vi "LSMcontroller_v66_improvedwfhandling.vi"() -> ()   [LabVIEW 2015] (continued)
                    n4209 = local read "Vy-max draw"() -> (w1158:dbl)
                    n4210 = local read "Vx-min draw"() -> (w1161:dbl)
                    n4211 = local read "Vx-max draw"() -> (w1160:dbl)
                    n4212 = local read "xpixels ref"() -> (w1157:i32)
                    n4213 = local read "ypixels ref"() -> (w1156:i32)
                    n4214 = local read "ROI Type"() -> (w1155:u16)
                    n4215 = local read "srateAODOtt"() -> (w1166:dbl)
                    n4216 = local read "# of frames"() -> (w1171:i32)
                    n4217 = local read "refreshtime"() -> (w1163:dbl)
                    n4218 = local read "Pel"() -> (w1154:dbl)
                    n4219 = local read "bin"() -> (w1169:dbl)
                    n4220 = local read "Override AI buffer"() -> (w1152:bool)
                    n4221 = local read "finite samples"() -> (w1178:bool)
                    n4222 = local read "srateAODOtt"() -> (w1165:dbl)
                    n4223 = local read "srateAODOtt"() -> (w1172:dbl)
                    n4224 = local read "continuous"() -> (w1177:bool)
                    n4225 = local read "Angle ref"() -> (w1162:dbl)
                    n4226 = local read "wavdet"() -> (w1179:bool)
                    n4227 = local read "Vx-ref"() -> (w1174:dbl)
                    n4228 = local read "Vy-ref"() -> (w1176:dbl)
                    n4229 = local read "avpp"() -> (w1175:i32)
                    n4230 = call "tt_timeandsamples.vi"("bin"=w1169, "refreshtime"=w1163, "srateAODOtt"=w1166, "tot#ofsamples"=w1171) -> ("refreshrate"=w1167:dbl, "refreshbuffer"=w1168:i32, "timetracecycles"=w1173:i32)  [unwired: 5 in]
                    n4231 = local read "bin"() -> (w1170:dbl)
                    n4232 = call "2pparameters.vi"("command"="get") -> ("params out"=w1182:T10)  [unwired: 1 in]
                    n4233 = Bundle By Name(cluster=w1182, "Drawing Mode"=w1155, "measpoints"=w1171, "tt_cycles"=w1173, "refreshbuffer"=w1168, "refreshrate"=w1167, "Vx-ref"=w1174, "Vy-ref"=w1176, "srate"=w1165, "finite"=w1178, "cont"=w1177, "wavdet"=w1179, "avpp"=w1175, "srateAODO"=w1172, "bufferAI"=w1168, "bin"=w1170, "Angle Img"=w1162, "Vxminref"=w1161, "Vxmaxref"=w1160, "Vyminref"=w1159, "Vymaxref"=w1158, "Xpixels Img"=w1157, "Ypixels Img"=w1156, "Pel"=w1154, "Vz-reset"=0.0, "AIoverride"=w1152, "type"="Timetrace") -> (w1180:T10)
                    n4234 = Reciprocal(x=w1167) -> (1/x=w1164:dbl)
                    n4235 = local write "refreshtime"(w1164) -> ()
                    n4236 = call "2pparameters.vi"("Params in"=w1180, "command"="set") -> ()  [unwired: 1 out]
                  }
                  frame "Lifetime (point)" {
                  }
                }
              }
              frame #1 {
                w1185 = FALSE ("wavdet")
                n4237 = call "2pparameters.vi"("command"="get") -> ("params out"=w1189:T10)  [unwired: 1 in]
                n4238 = Bundle By Name(cluster=w1189, "finite"=w1185, "cont"=w1185, "wavdet"=TRUE) -> (w1186:T10)
                n4239 = call "2pparameters.vi"("Params in"=w1186, "command"="set") -> ()  [unwired: 1 out]
              }
              frame #2 {
                n4240 = local read "Meastab"() -> (w1194:enum32{"X-Y Image", "Linescan", "Timetrace"})
                n4241 = property on="refwf" class="Ring (strict)"() -> ("RingText.Text"=w1197:string)  [unwired: 2 in, 2 out]
                n4242 = case shown="\"Timetrace\"" w1194 {
                  tunnel: [w1207 w1208] -> w1193
                  frame "X-Y Image", Default {
                    n4243 = local read "Sampling rate"() -> (w1207:dbl)
                  }
                  frame "Timetrace" {
                    n4244 = local read "srateAODOtt"() -> (w1208:dbl)
                  }
                }
                n4245 = call "waveformsAObuffer.vi"("command"="get") -> ("AO wf out"=w1206:waveform(dbl)[])  [unwired: 1 in]
                n4246 = local read "wavdet"() -> (w1196:bool)
                n4247 = call "waveformsDObuffer.vi"("command"="get") -> ("DO wf out"=w1202:digitalwaveform[])  [unwired: 1 in]
                n4248 = call "correctwaveformsizetemp.vi"("new sampling frequency (Hz)"=w1193, "start"=FALSE, "reference waveforms to"=w1197, "Analog waveforms in"=w1206, "stop"=FALSE, "Digital waveforms in"=w1202) -> ("analog wf out"=w1200:waveform(dbl)[], "Digital wf out"=w1198:digitalwaveform[], "measpoints"=w1195:i32)
                n4249 = local write "Analog Lines Plot"(w1200) -> ()
                n4250 = call "GetNumCamFramesv2.vi"("Digital Waveform Graph"=w1198) -> ("Numeric"=w1199:i32)  [unwired: 10 in]
                n4251 = local write "Digital Lines Plot"(w1198) -> ()
                n4252 = call "waveformsDObuffer.vi"("DO wf in"=w1198, "command"="set") -> ()  [unwired: 1 out]
                n4253 = call "waveformsAObuffer.vi"("AO wf in"=w1200, "command"="set") -> ()  [unwired: 1 out]
                n4254 = local write "Total Camera Frames"(w1199) -> ()
                n4255 = case shown="True" w1196 {
                  tunnel: w1195 -> [_ w1209]
                  frame False {
                  }
                  frame True {
                    n4256 = local write "# of frames"(w1209) -> ()
                  }
                }
              }
              frame #3 {
                n4257 = local read "finite samples"() -> (w1210:bool)
                n4258 = local read "continuous"() -> (w1211:bool)
                n4259 = local read "wavdet"() -> (w1212:bool)
                n4260 = call "2pparameters.vi"("command"="get") -> ("params out"=w1215:T10)  [unwired: 1 in]
                n4261 = Bundle By Name(cluster=w1215, "finite"=w1210, "cont"=w1211, "wavdet"=w1212) -> (w1213:T10)
                n4262 = call "2pparameters.vi"("Params in"=w1213, "command"="set") -> ()  [unwired: 1 out]
              }
            }
          }
          event "load changed AOsq": Value Change {
            n4263 = event-data() -> ("NewVal"=w1217:bool)  [unwired: 1 in, 5 out]
            n4264 = case shown="True" w1217 {
              frame False {
              }
              frame True {
                n4265 = stacked-sequence {
                  seq-local: [_ _ _ w1359 _ _] -> [_ _ _ _ w1384 _]
                  seq-local: [_ _ _ w1358 _ _] -> [_ _ _ _ w1383 _]
                  seq-local: [_ _ w1325 _ _ _] -> [_ _ _ w1357 w1382 w1413]
                  frame #0 {
                    n4266 = local read "Measurement"() -> (w1219:T4)
                    n4267 = local write "changeAOsq"(TRUE ("addAO")) -> ()
                    n4268 = case shown="\"X-Y-t movie\", Default" w1219 {
                      frame "X-Y-t movie", Default {
                        n4269 = local read "avpp"() -> (w1240:i32)
                        n4270 = local read "Angle ref"() -> (w1239:dbl)
                        n4271 = local read "ROI Type"() -> (w1238:u16)
                        n4272 = local read "xpixels ref"() -> (w1235:i32)
                        n4273 = local read "Vx-min ref"() -> (w1234:dbl)
                        n4274 = local read "Vx-max ref"() -> (w1233:dbl)
                        n4275 = local read "ypixels ref"() -> (w1231:i32)
                        n4276 = local read "Vy-min ref"() -> (w1232:dbl)
                        n4277 = local read "Vy-max ref"() -> (w1228:dbl)
                        n4278 = local read "Sampling rate"() -> (w1222:dbl)
                        n4279 = local read "finite samples"() -> (w1223:bool)
                        n4280 = local read "continuous"() -> (w1226:bool)
                        n4281 = local read "wavdet"() -> (w1227:bool)
                        n4282 = local read "# of frames"() -> (w1225:i32)
                        n4283 = local read "maxbufferAI"() -> (w1224:i32)
                        n4284 = local read "Override AI buffer"() -> (w1220:bool)
                        n4285 = call "2pparameters.vi"("command"="get") -> ("params out"=w1237:T10)  [unwired: 1 in]
                        n4286 = Bundle By Name(cluster=w1237, "type"="X-Y-t movie", "avpp"=w1240, "Angle Img"=w1239, "Xpixels Img"=w1235, "Vx-min Img"=w1234, "VX-max Img"=w1233, "Ypixels Img"=w1231, "Vy-min Img"=w1232, "Vy-max Img"=w1228, "srate"=w1222, "srate Img"=w1222, "finite"=w1223, "cont"=w1226, "wavdet"=w1227, "measpoints"=w1225, "maxbufferAI"=w1224, "Drawing Mode"=w1238, "Vz-reset"=0.0, "AIoverride"=w1220) -> (w1229:T10)
                        n4287 = call "2pparameters.vi"("Params in"=w1229, "command"="set") -> ()  [unwired: 1 out]
                      }
                      frame "X-Y-Z stack" {
                        n4288 = call "2pparameters.vi"("command"="get") -> ("params out"=w1244:T10)  [unwired: 1 in]
                        n4289 = Bundle By Name(cluster=w1244, "type"="X-Y-Z stack") -> (w1242:T10)
                        n4290 = call "2pparameters.vi"("Params in"=w1242, "command"="set") -> ()  [unwired: 1 out]
                      }
                      frame "Lifetime (scan)" {
                        n4291 = call "2pparameters.vi"("command"="get") -> ("params out"=w1249:T10)  [unwired: 1 in]
                        n4292 = Bundle By Name(cluster=w1249, "type"="Lifetime (scan)") -> (w1247:T10)
                        n4293 = call "2pparameters.vi"("Params in"=w1247, "command"="set") -> ()  [unwired: 1 out]
                      }
                      frame "Lifetime (contour)" {
                        n4294 = local read "Vy-min draw"() -> (w1259:dbl)
                        n4295 = local read "Vy-max draw"() -> (w1258:dbl)
                        n4296 = local read "Vx-min draw"() -> (w1261:dbl)
                        n4297 = local read "Vx-max draw"() -> (w1260:dbl)
                        n4298 = local read "xpixels ref"() -> (w1257:i32)
                        n4299 = local read "ypixels ref"() -> (w1256:i32)
                        n4300 = local read "ROI Type"() -> (w1255:u16)
                        n4301 = local read "srateAODOtt"() -> (w1266:dbl)
                        n4302 = local read "# of frames"() -> (w1271:i32)
                        n4303 = local read "refreshtime"() -> (w1263:dbl)
                        n4304 = local read "Pel"() -> (w1254:dbl)
                        n4305 = local read "bin"() -> (w1269:dbl)
                        n4306 = local read "Override AI buffer"() -> (w1252:bool)
                        n4307 = local read "finite samples"() -> (w1278:bool)
                        n4308 = local read "srateAODOtt"() -> (w1265:dbl)
                        n4309 = local read "srateAODOtt"() -> (w1272:dbl)
                        n4310 = local read "continuous"() -> (w1277:bool)
                        n4311 = local read "Angle ref"() -> (w1262:dbl)
                        n4312 = local read "wavdet"() -> (w1279:bool)
                        n4313 = local read "Vx-ref"() -> (w1274:dbl)
                        n4314 = local read "Vy-ref"() -> (w1276:dbl)
                        n4315 = local read "avpp"() -> (w1275:i32)
                        n4316 = call "tt_timeandsamples.vi"("bin"=w1269, "refreshtime"=w1263, "srateAODOtt"=w1266, "tot#ofsamples"=w1271) -> ("refreshrate"=w1267:dbl, "refreshbuffer"=w1268:i32, "timetracecycles"=w1273:i32)  [unwired: 5 in]
                        n4317 = local read "bin"() -> (w1270:dbl)
                        n4318 = call "2pparameters.vi"("command"="get") -> ("params out"=w1282:T10)  [unwired: 1 in]
                        n4319 = Bundle By Name(cluster=w1282, "Drawing Mode"=w1255, "measpoints"=w1271, "tt_cycles"=w1273, "refreshbuffer"=w1268, "refreshrate"=w1267, "Vx-ref"=w1274, "Vy-ref"=w1276, "srate"=w1265, "finite"=w1278, "cont"=w1277, "wavdet"=w1279, "avpp"=w1275, "srateAODO"=w1272, "bufferAI"=w1268, "bin"=w1270, "Angle Img"=w1262, "Vxminref"=w1261, "Vxmaxref"=w1260, "Vyminref"=w1259, "Vymaxref"=w1258, "Xpixels Img"=w1257, "Ypixels Img"=w1256, "Pel"=w1254, "Vz-reset"=0.0, "AIoverride"=w1252, "type"="Lifetime (contour)") -> (w1280:T10)
                        n4320 = Reciprocal(x=w1267) -> (1/x=w1264:dbl)
                        n4321 = local write "refreshtime"(w1264) -> ()
                        n4322 = call "2pparameters.vi"("Params in"=w1280, "command"="set") -> ()  [unwired: 1 out]
                      }
                      frame "X-Y-Z-t movie" {
                      }
                      frame "linescan" {
                      }
                      frame "Timetrace" {
                        n4323 = local read "Vy-min draw"() -> (w1292:dbl)
                        n4324 = local read "Vy-max draw"() -> (w1291:dbl)
                        n4325 = local read "Vx-min draw"() -> (w1294:dbl)
                        n4326 = local read "Vx-max draw"() -> (w1293:dbl)
                        n4327 = local read "xpixels ref"() -> (w1290:i32)
                        n4328 = local read "ypixels ref"() -> (w1289:i32)
                        n4329 = local read "ROI Type"() -> (w1288:u16)
                        n4330 = local read "srateAODOtt"() -> (w1299:dbl)
                        n4331 = local read "# of frames"() -> (w1304:i32)
                        n4332 = local read "refreshtime"() -> (w1296:dbl)
                        n4333 = local read "Pel"() -> (w1287:dbl)
                        n4334 = local read "bin"() -> (w1302:dbl)
                        n4335 = local read "Override AI buffer"() -> (w1285:bool)
                        n4336 = local read "finite samples"() -> (w1311:bool)
                        n4337 = local read "srateAODOtt"() -> (w1298:dbl)
                        n4338 = local read "srateAODOtt"() -> (w1305:dbl)
                        n4339 = local read "continuous"() -> (w1310:bool)
                        n4340 = local read "Angle ref"() -> (w1295:dbl)
                        n4341 = local read "wavdet"() -> (w1312:bool)
                        n4342 = local read "Vx-ref"() -> (w1307:dbl)
                        n4343 = local read "Vy-ref"() -> (w1309:dbl)
                        n4344 = local read "avpp"() -> (w1308:i32)
                        n4345 = call "tt_timeandsamples.vi"("bin"=w1302, "refreshtime"=w1296, "srateAODOtt"=w1299, "tot#ofsamples"=w1304) -> ("refreshrate"=w1300:dbl, "refreshbuffer"=w1301:i32, "timetracecycles"=w1306:i32)  [unwired: 5 in]
                        n4346 = local read "bin"() -> (w1303:dbl)
                        n4347 = call "2pparameters.vi"("command"="get") -> ("params out"=w1315:T10)  [unwired: 1 in]
                        n4348 = Bundle By Name(cluster=w1315, "Drawing Mode"=w1288, "measpoints"=w1304, "tt_cycles"=w1306, "refreshbuffer"=w1301, "refreshrate"=w1300, "Vx-ref"=w1307, "Vy-ref"=w1309, "srate"=w1298, "finite"=w1311, "cont"=w1310, "wavdet"=w1312, "avpp"=w1308, "srateAODO"=w1305, "bufferAI"=w1301, "bin"=w1303, "Angle Img"=w1295, "Vxminref"=w1294, "Vxmaxref"=w1293, "Vyminref"=w1292, "Vymaxref"=w1291, "Xpixels Img"=w1290, "Ypixels Img"=w1289, "Pel"=w1287, "Vz-reset"=0.0, "AIoverride"=w1285, "type"="Timetrace") -> (w1313:T10)
                        n4349 = Reciprocal(x=w1300) -> (1/x=w1297:dbl)
                        n4350 = local write "refreshtime"(w1297) -> ()
                        n4351 = call "2pparameters.vi"("Params in"=w1313, "command"="set") -> ()  [unwired: 1 out]
                      }
                      frame "Lifetime (point)" {
                      }
                    }
                  }
                  frame #1 {
                    w1318 = FALSE ("wavdet")
                    n4352 = call "2pparameters.vi"("command"="get") -> ("params out"=w1322:T10)  [unwired: 1 in]
                    n4353 = Bundle By Name(cluster=w1322, "finite"=w1318, "cont"=w1318, "wavdet"=TRUE) -> (w1319:T10)
                    n4354 = call "2pparameters.vi"("Params in"=w1319, "command"="set") -> ()  [unwired: 1 out]
                  }
                  frame #2 {
                    n4355 = local read "Meastab"() -> (w1349:enum32{"X-Y Image", "Linescan", "Timetrace"})
                    n4356 = property on="AO channels" class="Ring (strict)"() -> ("RingText.Text"=w1324:string)  [unwired: 2 in, 2 out]
                    n4357 = property on="refwf" class="Ring (strict)"() -> ("RingText.Text"=w1348:string)  [unwired: 2 in, 2 out]
                    n4358 = local read "Build analog waveform tabs"() -> (w1347:enum32{"Square", "Triangle", "Matlab"})
                    n4359 = case shown="\"X-Y Image\", Default" w1349 {
                      tunnel: [w1355 w1356] -> w1346
                      frame "X-Y Image", Default {
                        n4360 = local read "Sampling rate"() -> (w1355:dbl)
                      }
                      frame "Timetrace" {
                        n4361 = local read "srateAODOtt"() -> (w1356:dbl)
                      }
                    }
                    n4362 = local read "Matlab waveform path"() -> (w1339:path)
                    n4363 = local read "Period (ms)"() -> (w1342:dbl)
                    n4364 = local read "Frequency"() -> (w1341:dbl)
                    n4365 = local read "Tri Repeats"() -> (w1340:dbl)
                    n4366 = local read "Repeats"() -> (w1345:dbl)
                    n4367 = local read "Cycles"() -> (w1344:dbl)
                    n4368 = local read "Pulses"() -> (w1343:dbl)
                    n4369 = call "matlabwfexistsdialogue.vi"("Matlab waveform path"=w1339) -> ("mtalab waveform path out"=w1338:path)
                    n4370 = call "wfsizecalc.vi"("Sampling frequency (Hz)"=w1346, "AOtab"=w1347, "reference waveforms to"=w1348, "channel"=w1324, "Repeats"=w1345, "Cycles"=w1344, "Matlab wave file"=w1338, "pulses"=w1343, "Period (ms)"=w1342, "Frequency"=w1341, "Tri Repeats"=w1340) -> ("total size GB"=w1333:dbl, "gigabytesize wf"=w1329:dbl)  [unwired: 3 in]
                    n4371 = Greater?(x=w1329, y=0.5) -> (0:w1330:bool)
                    n4372 = Number To Fractional String(number=w1329, width (-)=i16 3) -> (F-format string=w1335:string)  [unwired: 2 in]
                    n4373 = Number To Fractional String(number=w1333, width (-)=i16 4) -> (F-format string=w1334:string)  [unwired: 2 in]
                    n4374 = Concatenate Strings("this is a crude approximation:\nyou're about to create a  " ("message"), w1335, " GB waveform for a total of " ("string"), w1334, " GB. Are you sure?" ("string")) -> (w1331:string)
                    n4375 = case shown="True" w1330 {
                      tunnel: w1331 -> [_ w1354]
                      tunnel: [TRUE ("T button?") w1351] -> w1325
                      frame False {
                      }
                      frame True {
                        n4376 = Two Button Dialog(message=w1354, 1:"No, don't do this." ("Center Button Text (\"No\")"), 2:"Yes, continue. " ("Left Button Text (\"Yes\")")) -> (T button?=w1351:bool)
                      }
                    }
                  }
                  frame #3 {
                    n4377 = case shown="True" w1357 {
                      tunnel: [_ w1361] -> w1359
                      tunnel: [_ w1360] -> w1358
                      frame False {
                      }
                      frame True {
                        n4378 = local read "AO channels"() -> (w1363:u32)
                        n4379 = call "2pparameters.vi"("command"="get") -> ("params out"=w1365:T10)  [unwired: 1 in]
                        n4380 = Unbundle By Name(w1365) -> ("aAO"=w1364:u32[])
                        n4381 = Search 1D Array(1D array=w1364, element=w1363) -> (index of element=w1361:i32)  [unwired: 1 in]
                        n4382 = Greater?(x=w1361, y=-1) -> (0:w1360:bool)
                        n4383 = case shown="True" w1360 {
                          tunnel: w1361 -> [_ w1379]
                          frame False {
                          }
                          frame True {
                            n4384 = local read "Meastab"() -> (w1368:enum32{"X-Y Image", "Linescan", "Timetrace"})
                            n4385 = case shown="\"Timetrace\"" w1368 {
                              tunnel: [w1380 w1381] -> w1367
                              frame "X-Y Image", Default {
                                n4386 = local read "Sampling rate"() -> (w1380:dbl)
                              }
                              frame "Timetrace" {
                                n4387 = local read "srateAODOtt"() -> (w1381:dbl)
                              }
                            }
                            n4388 = local read "Start amplitude (V)"() -> (w1376:dbl)
                            n4389 = local read "phase shift (ms)"() -> (w1371:dbl)
                            n4390 = local read "Step size (V)"() -> (w1374:dbl)
                            n4391 = local read "Baseline (V)"() -> (w1375:dbl)
                            n4392 = local read "Period (ms)"() -> (w1372:dbl)
                            n4393 = local read "padding value"() -> (w1369:dbl)
                            n4394 = local read "Repeats"() -> (w1378:dbl)
                            n4395 = local read "Cycles"() -> (w1377:dbl)
                            n4396 = local read "DC (%)"() -> (w1373:dbl)
                            n4397 = local read "Pulses"() -> (w1370:dbl)
                            n4398 = call "replace AO square wf param.vi"("Baseline (V)"=w1375, "Start amplitude (V)"=w1376, "Cycles"=w1377, "Repeats"=w1378, "index of AO wave"=w1379, "Step size (V)"=w1374, "DC (%)"=w1373, "Sampling frequency (Hz)"=w1367, "Period (ms)"=w1372, "Cycle length (s)"=w1371, "Pulses"=w1370, "padding value"=w1369) -> ()  [unwired: 4 in]
                          }
                        }
                      }
                    }
                  }
                  frame #4 {
                    n4399 = case shown="True" w1382 {
                      tunnel: w1384 -> [_ w1386]
                      tunnel: w1383 -> [_ w1385]
                      frame False {
                      }
                      frame True {
                        n4400 = case shown="True" w1385 {
                          tunnel: w1386 -> [_ w1394]
                          frame False {
                          }
                          frame True {
                            n4401 = call "waveformparamsv2.vi"("command"="get") -> ("Params out"=w1408:T14)  [unwired: 4 in, 2 out]
                            n4402 = Unbundle By Name(w1408) -> ("AO parameters"=w1407:T15)
                            n4403 = local read "Meastab"() -> (w1389:enum32{"X-Y Image", "Linescan", "Timetrace"})
                            n4404 = case shown="\"Timetrace\"" w1389 {
                              tunnel: [w1410 w1411] -> w1398
                              frame "X-Y Image", Default {
                                n4405 = local read "Sampling rate"() -> (w1410:dbl)
                              }
                              frame "Timetrace" {
                                n4406 = local read "srateAODOtt"() -> (w1411:dbl)
                              }
                            }
                            n4407 = Index Array(array=w1407, index=w1394) -> (element=w1396:T16)
                            n4408 = call "waveformsAObuffer.vi"("command"="get") -> ("AO wf out"=w1395:waveform(dbl)[])  [unwired: 1 in]
                            n4409 = call "generateRampedSquareWave_fromAOparameters.vi"("AO params"=w1396) -> ("Waveform"=w1393:waveform(dbl))  [unwired: 1 out]
                            n4410 = property on="refwf" class="Ring (strict)"() -> ("RingText.Text"=w1397:string)  [unwired: 2 in, 2 out]
                            n4411 = Replace Array Subset(array=w1395, new element=w1393, index=w1394) -> (w1392:waveform(dbl)[])
                            n4412 = call "waveformsDObuffer.vi"("command"="get") -> ("DO wf out"=w1403:digitalwaveform[])  [unwired: 1 in]
                            n4413 = call "correctwaveformsizetemp.vi"("new sampling frequency (Hz)"=w1398, "start"=FALSE, "reference waveforms to"=w1397, "Analog waveforms in"=w1392, "stop"=FALSE, "Digital waveforms in"=w1403) -> ("analog wf out"=w1401:waveform(dbl)[], "Digital wf out"=w1399:digitalwaveform[], "measpoints"=w1390:i32)
                            n4414 = local read "wavdet"() -> (w1391:bool)
                            n4415 = local write "Analog Lines Plot"(w1401) -> ()
                            n4416 = call "GetNumCamFramesv2.vi"("Digital Waveform Graph"=w1399) -> ("Numeric"=w1400:i32)  [unwired: 10 in]
                            n4417 = local write "Digital Lines Plot"(w1399) -> ()
                            n4418 = call "waveformsAObuffer.vi"("AO wf in"=w1401, "command"="set") -> ()  [unwired: 1 out]
                            n4419 = call "waveformsDObuffer.vi"("DO wf in"=w1399, "command"="set") -> ()  [unwired: 1 out]
                            n4420 = local write "Total Camera Frames"(w1400) -> ()
                            n4421 = case shown="True" w1391 {
                              tunnel: w1390 -> [_ w1412]
                              frame False {
                              }
                              frame True {
                                n4422 = local write "# of frames"(w1412) -> ()
                              }
                            }
                          }
                        }
                      }
                    }
                  }
                  frame #5 {
                    w1414 = FALSE ("addAO")
                    n4423 = local read "finite samples"() -> (w1415:bool)
                    n4424 = local read "continuous"() -> (w1416:bool)
                    n4425 = local read "wavdet"() -> (w1417:bool)
                    n4426 = local write "changeAOsq"(w1414) -> ()
                    n4427 = case shown="True" w1413 {
                      frame False {
                      }
                      frame True {
                        n4428 = local write "not loaded"(FALSE ("not loaded")) -> ()
                      }
                    }
                    n4429 = property on="load changed AOsq" class="Bool (strict)"("Val(Sgnl)"=w1414) -> ()  [unwired: 2 in, 2 out]
                    n4430 = call "2pparameters.vi"("command"="get") -> ("params out"=w1420:T10)  [unwired: 1 in]
                    n4431 = Bundle By Name(cluster=w1420, "finite"=w1415, "cont"=w1416, "wavdet"=w1417) -> (w1418:T10)
                    n4432 = call "2pparameters.vi"("Params in"=w1418, "command"="set") -> ()  [unwired: 1 out]
                  }
                }
              }
            }
          }
          event "load changed AOtri": Value Change {
            n4433 = event-data() -> ("NewVal"=w1423:bool)  [unwired: 1 in, 5 out]
            n4434 = case shown="True" w1423 {
              frame False {
              }
              frame True {
                n4435 = stacked-sequence {
                  seq-local: [_ _ _ w1565 _ _] -> [_ _ _ _ w1586 _]
                  seq-local: [_ _ _ w1564 _ _] -> [_ _ _ _ w1585 _]
                  seq-local: [_ _ w1531 _ _ _] -> [_ _ _ w1563 w1584 w1615]
                  frame #0 {
                    n4436 = local read "Measurement"() -> (w1425:T4)
                    n4437 = local write "changeAOtri"(TRUE ("addAO")) -> ()
                    n4438 = case shown="\"X-Y-t movie\", Default" w1425 {
                      frame "X-Y-t movie", Default {
                        n4439 = local read "avpp"() -> (w1446:i32)
                        n4440 = local read "Angle ref"() -> (w1445:dbl)
                        n4441 = local read "ROI Type"() -> (w1444:u16)
                        n4442 = local read "xpixels ref"() -> (w1441:i32)
                        n4443 = local read "Vx-min ref"() -> (w1440:dbl)
                        n4444 = local read "Vx-max ref"() -> (w1439:dbl)
                        n4445 = local read "ypixels ref"() -> (w1437:i32)
                        n4446 = local read "Vy-min ref"() -> (w1438:dbl)
                        n4447 = local read "Vy-max ref"() -> (w1434:dbl)
                        n4448 = local read "Sampling rate"() -> (w1428:dbl)
                        n4449 = local read "finite samples"() -> (w1429:bool)
                        n4450 = local read "continuous"() -> (w1432:bool)
                        n4451 = local read "wavdet"() -> (w1433:bool)
                        n4452 = local read "# of frames"() -> (w1431:i32)
                        n4453 = local read "maxbufferAI"() -> (w1430:i32)
                        n4454 = local read "Override AI buffer"() -> (w1426:bool)
                        n4455 = call "2pparameters.vi"("command"="get") -> ("params out"=w1443:T10)  [unwired: 1 in]
                        n4456 = Bundle By Name(cluster=w1443, "type"="X-Y-t movie", "avpp"=w1446, "Angle Img"=w1445, "Xpixels Img"=w1441, "Vx-min Img"=w1440, "VX-max Img"=w1439, "Ypixels Img"=w1437, "Vy-min Img"=w1438, "Vy-max Img"=w1434, "srate"=w1428, "srate Img"=w1428, "finite"=w1429, "cont"=w1432, "wavdet"=w1433, "measpoints"=w1431, "maxbufferAI"=w1430, "Drawing Mode"=w1444, "Vz-reset"=0.0, "AIoverride"=w1426) -> (w1435:T10)
                        n4457 = call "2pparameters.vi"("Params in"=w1435, "command"="set") -> ()  [unwired: 1 out]
                      }
                      frame "X-Y-Z stack" {
                        n4458 = call "2pparameters.vi"("command"="get") -> ("params out"=w1450:T10)  [unwired: 1 in]
                        n4459 = Bundle By Name(cluster=w1450, "type"="X-Y-Z stack") -> (w1448:T10)
                        n4460 = call "2pparameters.vi"("Params in"=w1448, "command"="set") -> ()  [unwired: 1 out]
                      }
                      frame "Lifetime (scan)" {
                        n4461 = call "2pparameters.vi"("command"="get") -> ("params out"=w1455:T10)  [unwired: 1 in]
                        n4462 = Bundle By Name(cluster=w1455, "type"="Lifetime (scan)") -> (w1453:T10)
                        n4463 = call "2pparameters.vi"("Params in"=w1453, "command"="set") -> ()  [unwired: 1 out]
                      }
                      frame "Lifetime (contour)" {
                        n4464 = local read "Vy-min draw"() -> (w1465:dbl)
                        n4465 = local read "Vy-max draw"() -> (w1464:dbl)
                        n4466 = local read "Vx-min draw"() -> (w1467:dbl)
                        n4467 = local read "Vx-max draw"() -> (w1466:dbl)
                        n4468 = local read "xpixels ref"() -> (w1463:i32)
                        n4469 = local read "ypixels ref"() -> (w1462:i32)
                        n4470 = local read "ROI Type"() -> (w1461:u16)
                        n4471 = local read "srateAODOtt"() -> (w1472:dbl)
                        n4472 = local read "# of frames"() -> (w1477:i32)
                        n4473 = local read "refreshtime"() -> (w1469:dbl)
                        n4474 = local read "Pel"() -> (w1460:dbl)
                        n4475 = local read "bin"() -> (w1475:dbl)
                        n4476 = local read "Override AI buffer"() -> (w1458:bool)
                        n4477 = local read "finite samples"() -> (w1484:bool)
                        n4478 = local read "srateAODOtt"() -> (w1471:dbl)
                        n4479 = local read "srateAODOtt"() -> (w1478:dbl)
                        n4480 = local read "continuous"() -> (w1483:bool)
                        n4481 = local read "Angle ref"() -> (w1468:dbl)
                        n4482 = local read "wavdet"() -> (w1485:bool)
                        n4483 = local read "Vx-ref"() -> (w1480:dbl)
                        n4484 = local read "Vy-ref"() -> (w1482:dbl)
                        n4485 = local read "avpp"() -> (w1481:i32)
                        n4486 = call "tt_timeandsamples.vi"("bin"=w1475, "refreshtime"=w1469, "srateAODOtt"=w1472, "tot#ofsamples"=w1477) -> ("refreshrate"=w1473:dbl, "refreshbuffer"=w1474:i32, "timetracecycles"=w1479:i32)  [unwired: 5 in]
                        n4487 = local read "bin"() -> (w1476:dbl)
                        n4488 = call "2pparameters.vi"("command"="get") -> ("params out"=w1488:T10)  [unwired: 1 in]
                        n4489 = Bundle By Name(cluster=w1488, "Drawing Mode"=w1461, "measpoints"=w1477, "tt_cycles"=w1479, "refreshbuffer"=w1474, "refreshrate"=w1473, "Vx-ref"=w1480, "Vy-ref"=w1482, "srate"=w1471, "finite"=w1484, "cont"=w1483, "wavdet"=w1485, "avpp"=w1481, "srateAODO"=w1478, "bufferAI"=w1474, "bin"=w1476, "Angle Img"=w1468, "Vxminref"=w1467, "Vxmaxref"=w1466, "Vyminref"=w1465, "Vymaxref"=w1464, "Xpixels Img"=w1463, "Ypixels Img"=w1462, "Pel"=w1460, "Vz-reset"=0.0, "AIoverride"=w1458, "type"="Lifetime (contour)") -> (w1486:T10)
                        n4490 = Reciprocal(x=w1473) -> (1/x=w1470:dbl)
                        n4491 = local write "refreshtime"(w1470) -> ()
                        n4492 = call "2pparameters.vi"("Params in"=w1486, "command"="set") -> ()  [unwired: 1 out]
                      }
                      frame "X-Y-Z-t movie" {
                      }
                      frame "linescan" {
                      }
                      frame "Timetrace" {
                        n4493 = local read "Vy-min draw"() -> (w1498:dbl)
                        n4494 = local read "Vy-max draw"() -> (w1497:dbl)
                        n4495 = local read "Vx-min draw"() -> (w1500:dbl)
                        n4496 = local read "Vx-max draw"() -> (w1499:dbl)
                        n4497 = local read "xpixels ref"() -> (w1496:i32)
                        n4498 = local read "ypixels ref"() -> (w1495:i32)
                        n4499 = local read "ROI Type"() -> (w1494:u16)
                        n4500 = local read "srateAODOtt"() -> (w1505:dbl)
                        n4501 = local read "# of frames"() -> (w1510:i32)
                        n4502 = local read "refreshtime"() -> (w1502:dbl)
                        n4503 = local read "Pel"() -> (w1493:dbl)
                        n4504 = local read "bin"() -> (w1508:dbl)
                        n4505 = local read "Override AI buffer"() -> (w1491:bool)
                        n4506 = local read "finite samples"() -> (w1517:bool)
                        n4507 = local read "srateAODOtt"() -> (w1504:dbl)
                        n4508 = local read "srateAODOtt"() -> (w1511:dbl)
                        n4509 = local read "continuous"() -> (w1516:bool)
                        n4510 = local read "Angle ref"() -> (w1501:dbl)
                        n4511 = local read "wavdet"() -> (w1518:bool)
                        n4512 = local read "Vx-ref"() -> (w1513:dbl)
                        n4513 = local read "Vy-ref"() -> (w1515:dbl)
                        n4514 = local read "avpp"() -> (w1514:i32)
                        n4515 = call "tt_timeandsamples.vi"("bin"=w1508, "refreshtime"=w1502, "srateAODOtt"=w1505, "tot#ofsamples"=w1510) -> ("refreshrate"=w1506:dbl, "refreshbuffer"=w1507:i32, "timetracecycles"=w1512:i32)  [unwired: 5 in]
                        n4516 = local read "bin"() -> (w1509:dbl)
                        n4517 = call "2pparameters.vi"("command"="get") -> ("params out"=w1521:T10)  [unwired: 1 in]
                        n4518 = Bundle By Name(cluster=w1521, "Drawing Mode"=w1494, "measpoints"=w1510, "tt_cycles"=w1512, "refreshbuffer"=w1507, "refreshrate"=w1506, "Vx-ref"=w1513, "Vy-ref"=w1515, "srate"=w1504, "finite"=w1517, "cont"=w1516, "wavdet"=w1518, "avpp"=w1514, "srateAODO"=w1511, "bufferAI"=w1507, "bin"=w1509, "Angle Img"=w1501, "Vxminref"=w1500, "Vxmaxref"=w1499, "Vyminref"=w1498, "Vymaxref"=w1497, "Xpixels Img"=w1496, "Ypixels Img"=w1495, "Pel"=w1493, "Vz-reset"=0.0, "AIoverride"=w1491, "type"="Timetrace") -> (w1519:T10)
                        n4519 = Reciprocal(x=w1506) -> (1/x=w1503:dbl)
                        n4520 = local write "refreshtime"(w1503) -> ()
                        n4521 = call "2pparameters.vi"("Params in"=w1519, "command"="set") -> ()  [unwired: 1 out]
                      }
                      frame "Lifetime (point)" {
                      }
                    }
                  }
                  frame #1 {
                    w1524 = FALSE ("wavdet")
                    n4522 = call "2pparameters.vi"("command"="get") -> ("params out"=w1528:T10)  [unwired: 1 in]
                    n4523 = Bundle By Name(cluster=w1528, "finite"=w1524, "cont"=w1524, "wavdet"=TRUE) -> (w1525:T10)
                    n4524 = call "2pparameters.vi"("Params in"=w1525, "command"="set") -> ()  [unwired: 1 out]
                  }
                  frame #2 {
                    n4525 = local read "Meastab"() -> (w1555:enum32{"X-Y Image", "Linescan", "Timetrace"})
                    n4526 = property on="AO channels" class="Ring (strict)"() -> ("RingText.Text"=w1530:string)  [unwired: 2 in, 2 out]
                    n4527 = property on="refwf" class="Ring (strict)"() -> ("RingText.Text"=w1554:string)  [unwired: 2 in, 2 out]
                    n4528 = local read "Build analog waveform tabs"() -> (w1553:enum32{"Square", "Triangle", "Matlab"})
                    n4529 = case shown="\"X-Y Image\", Default" w1555 {
                      tunnel: [w1561 w1562] -> w1552
                      frame "X-Y Image", Default {
                        n4530 = local read "Sampling rate"() -> (w1561:dbl)
                      }
                      frame "Timetrace" {
                        n4531 = local read "srateAODOtt"() -> (w1562:dbl)
                      }
                    }
                    n4532 = local read "Matlab waveform path"() -> (w1545:path)
                    n4533 = local read "Period (ms)"() -> (w1548:dbl)
                    n4534 = local read "Frequency"() -> (w1547:dbl)
                    n4535 = local read "Tri Repeats"() -> (w1546:dbl)
                    n4536 = local read "Repeats"() -> (w1551:dbl)
                    n4537 = local read "Cycles"() -> (w1550:dbl)
                    n4538 = local read "Pulses"() -> (w1549:dbl)
                    n4539 = call "matlabwfexistsdialogue.vi"("Matlab waveform path"=w1545) -> ("mtalab waveform path out"=w1544:path)
                    n4540 = call "wfsizecalc.vi"("Sampling frequency (Hz)"=w1552, "AOtab"=w1553, "reference waveforms to"=w1554, "channel"=w1530, "Repeats"=w1551, "Cycles"=w1550, "Matlab wave file"=w1544, "pulses"=w1549, "Period (ms)"=w1548, "Frequency"=w1547, "Tri Repeats"=w1546) -> ("total size GB"=w1539:dbl, "gigabytesize wf"=w1535:dbl)  [unwired: 3 in]
                    n4541 = Greater?(x=w1535, y=0.5) -> (0:w1536:bool)
                    n4542 = Number To Fractional String(number=w1535, width (-)=i16 3) -> (F-format string=w1541:string)  [unwired: 2 in]
                    n4543 = Number To Fractional String(number=w1539, width (-)=i16 4) -> (F-format string=w1540:string)  [unwired: 2 in]
                    n4544 = Concatenate Strings("this is a crude approximation:\nyou're about to create a  " ("message"), w1541, " GB waveform for a total of " ("string"), w1540, " GB. Are you sure?" ("string")) -> (w1537:string)
                    n4545 = case shown="True" w1536 {
                      tunnel: w1537 -> [_ w1560]
                      tunnel: [TRUE ("T button?") w1557] -> w1531
                      frame False {
                      }
                      frame True {
                        n4546 = Two Button Dialog(message=w1560, 1:"No, don't do this." ("Center Button Text (\"No\")"), 2:"Yes, continue. " ("Left Button Text (\"Yes\")")) -> (T button?=w1557:bool)
                      }
                    }
                  }
                  frame #3 {
                    n4547 = case shown="True" w1563 {
                      tunnel: [_ w1567] -> w1565
                      tunnel: [_ w1566] -> w1564
                      frame False {
                      }
                      frame True {
                        n4548 = local read "AO channels"() -> (w1569:u32)
                        n4549 = call "2pparameters.vi"("command"="get") -> ("params out"=w1571:T10)  [unwired: 1 in]
                        n4550 = Unbundle By Name(w1571) -> ("aAO"=w1570:u32[])
                        n4551 = Search 1D Array(1D array=w1570, element=w1569) -> (index of element=w1567:i32)  [unwired: 1 in]
                        n4552 = Greater?(x=w1567, y=-1) -> (0:w1566:bool)
                        n4553 = case shown="True" w1566 {
                          tunnel: w1567 -> [_ w1581]
                          frame False {
                          }
                          frame True {
                            n4554 = local read "Meastab"() -> (w1574:enum32{"X-Y Image", "Linescan", "Timetrace"})
                            n4555 = local read "Tri padding value"() -> (w1575:dbl)
                            n4556 = local read "Amplitude (V)"() -> (w1579:dbl)
                            n4557 = local read "Tri Phase (s)"() -> (w1576:dbl)
                            n4558 = local read "Tri Repeats"() -> (w1577:dbl)
                            n4559 = local read "Frequency"() -> (w1578:dbl)
                            n4560 = local read "Offset (V)"() -> (w1580:dbl)
                            n4561 = case shown="\"Timetrace\"" w1574 {
                              tunnel: [w1582 w1583] -> w1573
                              frame "X-Y Image", Default {
                                n4562 = local read "Sampling rate"() -> (w1582:dbl)
                              }
                              frame "Timetrace" {
                                n4563 = local read "srateAODOtt"() -> (w1583:dbl)
                              }
                            }
                            n4564 = call "replace AO tri wf param.vi"("padding value"=w1575, "index of AO wave"=w1581, "Tri phase"=w1576, "Sampling frequency (Hz)"=w1573, "Tri Repeats"=w1577, "Frequency"=w1578, "Amplitude (V)"=w1579, "Offset (V)"=w1580) -> ()
                          }
                        }
                      }
                    }
                  }
                  frame #4 {
                    n4565 = case shown="True" w1584 {
                      tunnel: w1586 -> [_ w1588]
                      tunnel: w1585 -> [_ w1587]
                      frame False {
                      }
                      frame True {
                        n4566 = case shown="True" w1587 {
                          tunnel: w1588 -> [_ w1597]
                          frame False {
                          }
                          frame True {
                            n4567 = call "waveformparamsv2.vi"("command"="get") -> ("Params out"=w1610:T14)  [unwired: 4 in, 2 out]
                            n4568 = Unbundle By Name(w1610) -> ("AO parameters"=w1609:T15)
                            n4569 = local read "Meastab"() -> (w1592:enum32{"X-Y Image", "Linescan", "Timetrace"})
                            n4570 = case shown="\"Timetrace\"" w1592 {
                              tunnel: [w1612 w1613] -> w1591
                              frame "X-Y Image", Default {
                                n4571 = local read "Sampling rate"() -> (w1612:dbl)
                              }
                              frame "Timetrace" {
                                n4572 = local read "srateAODOtt"() -> (w1613:dbl)
                              }
                            }
                            n4573 = Index Array(array=w1609, index=w1597) -> (element=w1599:T16)
                            n4574 = call "waveformsAObuffer.vi"("command"="get") -> ("AO wf out"=w1598:waveform(dbl)[])  [unwired: 1 in]
                            n4575 = call "generateTriWave_fromAOparameters.vi"("AO params"=w1599) -> ("Waveform"=w1596:waveform(dbl))  [unwired: 1 out]
                            n4576 = property on="refwf" class="Ring (strict)"() -> ("RingText.Text"=w1600:string)  [unwired: 2 in, 2 out]
                            n4577 = Replace Array Subset(array=w1598, new element=w1596, index=w1597) -> (w1595:waveform(dbl)[])
                            n4578 = call "waveformsDObuffer.vi"("command"="get") -> ("DO wf out"=w1605:digitalwaveform[])  [unwired: 1 in]
                            n4579 = call "correctwaveformsizetemp.vi"("new sampling frequency (Hz)"=w1591, "start"=FALSE, "reference waveforms to"=w1600, "Analog waveforms in"=w1595, "stop"=FALSE, "Digital waveforms in"=w1605) -> ("analog wf out"=w1603:waveform(dbl)[], "Digital wf out"=w1601:digitalwaveform[], "measpoints"=w1593:i32)
                            n4580 = local read "wavdet"() -> (w1594:bool)
                            n4581 = local write "Analog Lines Plot"(w1603) -> ()
                            n4582 = call "GetNumCamFramesv2.vi"("Digital Waveform Graph"=w1601) -> ("Numeric"=w1602:i32)  [unwired: 10 in]
                            n4583 = local write "Digital Lines Plot"(w1601) -> ()
                            n4584 = call "waveformsAObuffer.vi"("AO wf in"=w1603, "command"="set") -> ()  [unwired: 1 out]
                            n4585 = call "waveformsDObuffer.vi"("DO wf in"=w1601, "command"="set") -> ()  [unwired: 1 out]
                            n4586 = local write "Total Camera Frames"(w1602) -> ()
                            n4587 = case shown="True" w1594 {
                              tunnel: w1593 -> [_ w1614]
                              frame False {
                              }
                              frame True {
                                n4588 = local write "# of frames"(w1614) -> ()
                              }
                            }
                          }
                        }
                      }
                    }
                  }
                  frame #5 {
                    w1616 = FALSE ("addAO")
                    n4589 = case shown="True" w1615 {
                      frame False {
                      }
                      frame True {
                        n4590 = local write "not loadedtri"(FALSE ("not loadedtri")) -> ()
                      }
                    }
                    n4591 = local write "changeAOtri"(w1616) -> ()
                    n4592 = property on="load changed AOtri" class="Bool (strict)"("Val(Sgnl)"=w1616) -> ()  [unwired: 2 in, 2 out]
                    n4593 = local read "finite samples"() -> (w1617:bool)
                    n4594 = local read "continuous"() -> (w1618:bool)
                    n4595 = local read "wavdet"() -> (w1619:bool)
                    n4596 = call "2pparameters.vi"("command"="get") -> ("params out"=w1622:T10)  [unwired: 1 in]
                    n4597 = Bundle By Name(cluster=w1622, "finite"=w1617, "cont"=w1618, "wavdet"=w1619) -> (w1620:T10)
                    n4598 = call "2pparameters.vi"("Params in"=w1620, "command"="set") -> ()  [unwired: 1 out]
                  }
                }
              }
            }
          }
          event "Load Matlab Waveform": Value Change {
            n4599 = event-data() -> ("NewVal"=w1625:bool)  [unwired: 1 in, 5 out]
            n4600 = case shown="True" w1625 {
              frame False {
              }
              frame True {
                n4601 = stacked-sequence {
                  seq-local: [_ _ _ w1767 _ _] -> [_ _ _ _ w1785 _]
                  seq-local: [_ _ _ w1766 _ _] -> [_ _ _ _ w1784 _]
                  seq-local: [_ _ w1733 _ _ _] -> [_ _ _ w1765 w1783 w1814]
                  frame #0 {
                    n4602 = local read "Measurement"() -> (w1627:T4)
                    n4603 = case shown="\"X-Y-t movie\", Default" w1627 {
                      frame "X-Y-t movie", Default {
                        n4604 = local read "avpp"() -> (w1648:i32)
                        n4605 = local read "Angle ref"() -> (w1647:dbl)
                        n4606 = local read "ROI Type"() -> (w1646:u16)
                        n4607 = local read "xpixels ref"() -> (w1643:i32)
                        n4608 = local read "Vx-min ref"() -> (w1642:dbl)
                        n4609 = local read "Vx-max ref"() -> (w1641:dbl)
                        n4610 = local read "ypixels ref"() -> (w1639:i32)
                        n4611 = local read "Vy-min ref"() -> (w1640:dbl)
                        n4612 = local read "Vy-max ref"() -> (w1636:dbl)
                        n4613 = local read "Sampling rate"() -> (w1630:dbl)
                        n4614 = local read "finite samples"() -> (w1631:bool)
                        n4615 = local read "continuous"() -> (w1634:bool)
                        n4616 = local read "wavdet"() -> (w1635:bool)
                        n4617 = local read "# of frames"() -> (w1633:i32)
                        n4618 = local read "maxbufferAI"() -> (w1632:i32)
                        n4619 = local read "Override AI buffer"() -> (w1628:bool)
                        n4620 = call "2pparameters.vi"("command"="get") -> ("params out"=w1645:T10)  [unwired: 1 in]
                        n4621 = Bundle By Name(cluster=w1645, "type"="X-Y-t movie", "avpp"=w1648, "Angle Img"=w1647, "Xpixels Img"=w1643, "Vx-min Img"=w1642, "VX-max Img"=w1641, "Ypixels Img"=w1639, "Vy-min Img"=w1640, "Vy-max Img"=w1636, "srate"=w1630, "srate Img"=w1630, "finite"=w1631, "cont"=w1634, "wavdet"=w1635, "measpoints"=w1633, "maxbufferAI"=w1632, "Drawing Mode"=w1646, "Vz-reset"=0.0, "AIoverride"=w1628) -> (w1637:T10)
                        n4622 = call "2pparameters.vi"("Params in"=w1637, "command"="set") -> ()  [unwired: 1 out]
                      }
                      frame "X-Y-Z stack" {
                        n4623 = call "2pparameters.vi"("command"="get") -> ("params out"=w1652:T10)  [unwired: 1 in]
                        n4624 = Bundle By Name(cluster=w1652, "type"="X-Y-Z stack") -> (w1650:T10)
                        n4625 = call "2pparameters.vi"("Params in"=w1650, "command"="set") -> ()  [unwired: 1 out]
                      }
                      frame "Lifetime (scan)" {
                        n4626 = call "2pparameters.vi"("command"="get") -> ("params out"=w1657:T10)  [unwired: 1 in]
                        n4627 = Bundle By Name(cluster=w1657, "type"="Lifetime (scan)") -> (w1655:T10)
                        n4628 = call "2pparameters.vi"("Params in"=w1655, "command"="set") -> ()  [unwired: 1 out]
                      }
                      frame "Lifetime (contour)" {
                        n4629 = local read "Vy-min draw"() -> (w1667:dbl)
                        n4630 = local read "Vy-max draw"() -> (w1666:dbl)
                        n4631 = local read "Vx-min draw"() -> (w1669:dbl)
                        n4632 = local read "Vx-max draw"() -> (w1668:dbl)
                        n4633 = local read "xpixels ref"() -> (w1665:i32)
                        n4634 = local read "ypixels ref"() -> (w1664:i32)
                        n4635 = local read "ROI Type"() -> (w1663:u16)
                        n4636 = local read "srateAODOtt"() -> (w1674:dbl)
                        n4637 = local read "# of frames"() -> (w1679:i32)
                        n4638 = local read "refreshtime"() -> (w1671:dbl)
                        n4639 = local read "Pel"() -> (w1662:dbl)
                        n4640 = local read "bin"() -> (w1677:dbl)
                        n4641 = local read "Override AI buffer"() -> (w1660:bool)
                        n4642 = local read "finite samples"() -> (w1686:bool)
                        n4643 = local read "srateAODOtt"() -> (w1673:dbl)
                        n4644 = local read "srateAODOtt"() -> (w1680:dbl)
                        n4645 = local read "continuous"() -> (w1685:bool)
                        n4646 = local read "Angle ref"() -> (w1670:dbl)
                        n4647 = local read "wavdet"() -> (w1687:bool)
                        n4648 = local read "Vx-ref"() -> (w1682:dbl)
                        n4649 = local read "Vy-ref"() -> (w1684:dbl)
                        n4650 = local read "avpp"() -> (w1683:i32)
                        n4651 = call "tt_timeandsamples.vi"("bin"=w1677, "refreshtime"=w1671, "srateAODOtt"=w1674, "tot#ofsamples"=w1679) -> ("refreshrate"=w1675:dbl, "refreshbuffer"=w1676:i32, "timetracecycles"=w1681:i32)  [unwired: 5 in]
                        n4652 = local read "bin"() -> (w1678:dbl)
                        n4653 = call "2pparameters.vi"("command"="get") -> ("params out"=w1690:T10)  [unwired: 1 in]
                        n4654 = Bundle By Name(cluster=w1690, "Drawing Mode"=w1663, "measpoints"=w1679, "tt_cycles"=w1681, "refreshbuffer"=w1676, "refreshrate"=w1675, "Vx-ref"=w1682, "Vy-ref"=w1684, "srate"=w1673, "finite"=w1686, "cont"=w1685, "wavdet"=w1687, "avpp"=w1683, "srateAODO"=w1680, "bufferAI"=w1676, "bin"=w1678, "Angle Img"=w1670, "Vxminref"=w1669, "Vxmaxref"=w1668, "Vyminref"=w1667, "Vymaxref"=w1666, "Xpixels Img"=w1665, "Ypixels Img"=w1664, "Pel"=w1662, "Vz-reset"=0.0, "AIoverride"=w1660, "type"="Lifetime (contour)") -> (w1688:T10)
                        n4655 = Reciprocal(x=w1675) -> (1/x=w1672:dbl)
                        n4656 = local write "refreshtime"(w1672) -> ()
                        n4657 = call "2pparameters.vi"("Params in"=w1688, "command"="set") -> ()  [unwired: 1 out]
                      }
                      frame "X-Y-Z-t movie" {
                      }
                      frame "linescan" {
                      }
                      frame "Timetrace" {
                        n4658 = local read "Vy-min draw"() -> (w1700:dbl)
                        n4659 = local read "Vy-max draw"() -> (w1699:dbl)
                        n4660 = local read "Vx-min draw"() -> (w1702:dbl)
                        n4661 = local read "Vx-max draw"() -> (w1701:dbl)
                        n4662 = local read "xpixels ref"() -> (w1698:i32)
                        n4663 = local read "ypixels ref"() -> (w1697:i32)
                        n4664 = local read "ROI Type"() -> (w1696:u16)
                        n4665 = local read "srateAODOtt"() -> (w1707:dbl)
                        n4666 = local read "# of frames"() -> (w1712:i32)
                        n4667 = local read "refreshtime"() -> (w1704:dbl)
                        n4668 = local read "Pel"() -> (w1695:dbl)
                        n4669 = local read "bin"() -> (w1710:dbl)
                        n4670 = local read "Override AI buffer"() -> (w1693:bool)
                        n4671 = local read "finite samples"() -> (w1719:bool)
                        n4672 = local read "srateAODOtt"() -> (w1706:dbl)
                        n4673 = local read "srateAODOtt"() -> (w1713:dbl)
                        n4674 = local read "continuous"() -> (w1718:bool)
                        n4675 = local read "Angle ref"() -> (w1703:dbl)
                        n4676 = local read "wavdet"() -> (w1720:bool)
                        n4677 = local read "Vx-ref"() -> (w1715:dbl)
                        n4678 = local read "Vy-ref"() -> (w1717:dbl)
                        n4679 = local read "avpp"() -> (w1716:i32)
                        n4680 = call "tt_timeandsamples.vi"("bin"=w1710, "refreshtime"=w1704, "srateAODOtt"=w1707, "tot#ofsamples"=w1712) -> ("refreshrate"=w1708:dbl, "refreshbuffer"=w1709:i32, "timetracecycles"=w1714:i32)  [unwired: 5 in]
                        n4681 = local read "bin"() -> (w1711:dbl)
                        n4682 = call "2pparameters.vi"("command"="get") -> ("params out"=w1723:T10)  [unwired: 1 in]
                        n4683 = Bundle By Name(cluster=w1723, "Drawing Mode"=w1696, "measpoints"=w1712, "tt_cycles"=w1714, "refreshbuffer"=w1709, "refreshrate"=w1708, "Vx-ref"=w1715, "Vy-ref"=w1717, "srate"=w1706, "finite"=w1719, "cont"=w1718, "wavdet"=w1720, "avpp"=w1716, "srateAODO"=w1713, "bufferAI"=w1709, "bin"=w1711, "Angle Img"=w1703, "Vxminref"=w1702, "Vxmaxref"=w1701, "Vyminref"=w1700, "Vymaxref"=w1699, "Xpixels Img"=w1698, "Ypixels Img"=w1697, "Pel"=w1695, "Vz-reset"=0.0, "AIoverride"=w1693, "type"="Timetrace") -> (w1721:T10)
                        n4684 = Reciprocal(x=w1708) -> (1/x=w1705:dbl)
                        n4685 = local write "refreshtime"(w1705) -> ()
                        n4686 = call "2pparameters.vi"("Params in"=w1721, "command"="set") -> ()  [unwired: 1 out]
                      }
                      frame "Lifetime (point)" {
                      }
                    }
                    n4687 = local write "changeAOmatlab"(TRUE ("addAO")) -> ()
                  }
                  frame #1 {
                    w1726 = FALSE ("wavdet")
                    n4688 = call "2pparameters.vi"("command"="get") -> ("params out"=w1730:T10)  [unwired: 1 in]
                    n4689 = Bundle By Name(cluster=w1730, "finite"=w1726, "cont"=w1726, "wavdet"=TRUE) -> (w1727:T10)
                    n4690 = call "2pparameters.vi"("Params in"=w1727, "command"="set") -> ()  [unwired: 1 out]
                  }
                  frame #2 {
                    n4691 = local read "Meastab"() -> (w1757:enum32{"X-Y Image", "Linescan", "Timetrace"})
                    n4692 = property on="AO channels" class="Ring (strict)"() -> ("RingText.Text"=w1732:string)  [unwired: 2 in, 2 out]
                    n4693 = property on="refwf" class="Ring (strict)"() -> ("RingText.Text"=w1756:string)  [unwired: 2 in, 2 out]
                    n4694 = local read "Build analog waveform tabs"() -> (w1755:enum32{"Square", "Triangle", "Matlab"})
                    n4695 = case shown="\"X-Y Image\", Default" w1757 {
                      tunnel: [w1763 w1764] -> w1754
                      frame "X-Y Image", Default {
                        n4696 = local read "Sampling rate"() -> (w1763:dbl)
                      }
                      frame "Timetrace" {
                        n4697 = local read "srateAODOtt"() -> (w1764:dbl)
                      }
                    }
                    n4698 = local read "Matlab waveform path"() -> (w1747:path)
                    n4699 = local read "Period (ms)"() -> (w1750:dbl)
                    n4700 = local read "Frequency"() -> (w1749:dbl)
                    n4701 = local read "Tri Repeats"() -> (w1748:dbl)
                    n4702 = local read "Repeats"() -> (w1753:dbl)
                    n4703 = local read "Cycles"() -> (w1752:dbl)
                    n4704 = local read "Pulses"() -> (w1751:dbl)
                    n4705 = call "matlabwfexistsdialogue.vi"("Matlab waveform path"=w1747) -> ("mtalab waveform path out"=w1746:path)
                    n4706 = call "wfsizecalc.vi"("Sampling frequency (Hz)"=w1754, "AOtab"=w1755, "reference waveforms to"=w1756, "channel"=w1732, "Repeats"=w1753, "Cycles"=w1752, "Matlab wave file"=w1746, "pulses"=w1751, "Period (ms)"=w1750, "Frequency"=w1749, "Tri Repeats"=w1748) -> ("total size GB"=w1741:dbl, "gigabytesize wf"=w1737:dbl)  [unwired: 3 in]
                    n4707 = Greater?(x=w1737, y=0.5) -> (0:w1738:bool)
                    n4708 = Number To Fractional String(number=w1737, width (-)=i16 3) -> (F-format string=w1743:string)  [unwired: 2 in]
                    n4709 = Number To Fractional String(number=w1741, width (-)=i16 4) -> (F-format string=w1742:string)  [unwired: 2 in]
                    n4710 = Concatenate Strings("this is a crude approximation:\nyou're about to create a  " ("message"), w1743, " GB waveform for a total of " ("string"), w1742, " GB. Are you sure?" ("string")) -> (w1739:string)
                    n4711 = case shown="True" w1738 {
                      tunnel: w1739 -> [_ w1762]
                      tunnel: [TRUE ("T button?") w1759] -> w1733
                      frame False {
                      }
                      frame True {
                        n4712 = Two Button Dialog(message=w1762, 1:"No, don't do this." ("Center Button Text (\"No\")"), 2:"Yes, continue. " ("Left Button Text (\"Yes\")")) -> (T button?=w1759:bool)
                      }
                    }
                  }
                  frame #3 {
                    n4713 = case shown="True" w1765 {
                      tunnel: [_ w1769] -> w1767
                      tunnel: [_ w1768] -> w1766
                      frame False {
                      }
                      frame True {
                        n4714 = local read "AO channels"() -> (w1771:u32)
                        n4715 = call "2pparameters.vi"("command"="get") -> ("params out"=w1773:T10)  [unwired: 1 in]
                        n4716 = Unbundle By Name(w1773) -> ("aAO"=w1772:u32[])
                        n4717 = Search 1D Array(1D array=w1772, element=w1771) -> (index of element=w1769:i32)  [unwired: 1 in]
                        n4718 = Greater?(x=w1769, y=-1) -> (0:w1768:bool)
                        n4719 = case shown="True" w1768 {
                          tunnel: w1769 -> [_ w1780]
                          frame False {
                          }
                          frame True {
                            n4720 = local read "Meastab"() -> (w1776:enum32{"X-Y Image", "Linescan", "Timetrace"})
                            n4721 = local read "Matlab waveform path"() -> (w1778:path)
                            n4722 = local read "Matlab padding value"() -> (w1779:dbl)
                            n4723 = case shown="\"Timetrace\"" w1776 {
                              tunnel: [w1781 w1782] -> w1775
                              frame "X-Y Image", Default {
                                n4724 = local read "Sampling rate"() -> (w1781:dbl)
                              }
                              frame "Timetrace" {
                                n4725 = local read "srateAODOtt"() -> (w1782:dbl)
                              }
                            }
                            n4726 = call "matlabwfexistsdialogue.vi"("Matlab waveform path"=w1778) -> ("mtalab waveform path out"=w1777:path)
                            n4727 = call "replace AO matlab param.vi"("Sampling frequency (Hz)"=w1775, "matlab wave file"=w1777, "index of AO wave"=w1780, "padding value"=w1779) -> ()  [unwired: 7 in]
                          }
                        }
                      }
                    }
                  }
                  frame #4 {
                    n4728 = case shown="True" w1783 {
                      tunnel: w1785 -> [_ w1787]
                      tunnel: w1784 -> [_ w1786]
                      frame False {
                      }
                      frame True {
                        n4729 = case shown="True" w1786 {
                          tunnel: w1787 -> [_ w1794]
                          frame False {
                          }
                          frame True {
                            n4730 = local read "Meastab"() -> (w1791:enum32{"X-Y Image", "Linescan", "Timetrace"})
                            n4731 = call "waveformparamsv2.vi"("command"="get") -> ("Params out"=w1797:T14)  [unwired: 4 in, 2 out]
                            n4732 = Unbundle By Name(w1797) -> ("AO parameters"=w1796:T15)
                            n4733 = case shown="\"Timetrace\"" w1791 {
                              tunnel: [w1811 w1812] -> w1790
                              frame "X-Y Image", Default {
                                n4734 = local read "Sampling rate"() -> (w1811:dbl)
                              }
                              frame "Timetrace" {
                                n4735 = local read "srateAODOtt"() -> (w1812:dbl)
                              }
                            }
                            n4736 = Index Array(array=w1796, index=w1794) -> (element=w1795:T16)
                            n4737 = call "waveformsAObuffer.vi"("command"="get") -> ("AO wf out"=w1801:waveform(dbl)[])  [unwired: 1 in]
                            n4738 = call "matlabAOwffromparam.vi"("Cluster"=w1795) -> ("Waveform"=w1799:waveform(dbl))  [unwired: 1 out]
                            n4739 = property on="refwf" class="Ring (strict)"() -> ("RingText.Text"=w1802:string)  [unwired: 2 in, 2 out]
                            n4740 = Replace Array Subset(array=w1801, new element=w1799, index=w1794) -> (w1800:waveform(dbl)[])
                            n4741 = call "waveformsDObuffer.vi"("command"="get") -> ("DO wf out"=w1807:digitalwaveform[])  [unwired: 1 in]
